vi "test2-ProcessSyncMessageInCSMLoop(SendAndReceive).vi"(8 "error in (no error)":errorcluster, 11 "TestCase in":refnum<class "testcase-CSMAddonLoopSupport.lvclass">) -> (0 "error out":errorcluster, 3 "TestCase out":refnum<class "testcase-CSMAddonLoopSupport.lvclass">)   [LabVIEW 2017, in "testcase-CSMAddonLoopSupport.lvclass"]
uses:
  testcase-CSMAddonLoopSupport.lvclass
  4585ddd5-ba69-4fd4-94fe-207595864cbd.vi
  a7620e19-6451-46a1-85ca-ade5edb58587.vi
  55fec5d7-cd22-46f7-b641-2c7c49619fc8.vi
  9cfd6824-310a-46c9-9b98-3854de5c7aa2.vi
  <vilib>/addons/_JKI Toolkits/VI Tester/TestCase.llb/TestCase.lvclass
  src/user.lib/_NEVSTOP/Communicable State Machine(CSM)/Communicable State Machine.lvlib
  C:/Program Files (x86)/National Instruments/LabVIEW 2017/vi.lib/addons/_JKI Toolkits/VI Tester/TestCase.llb/TestCase.lvclass
panel:
  out "LoopCount":i32
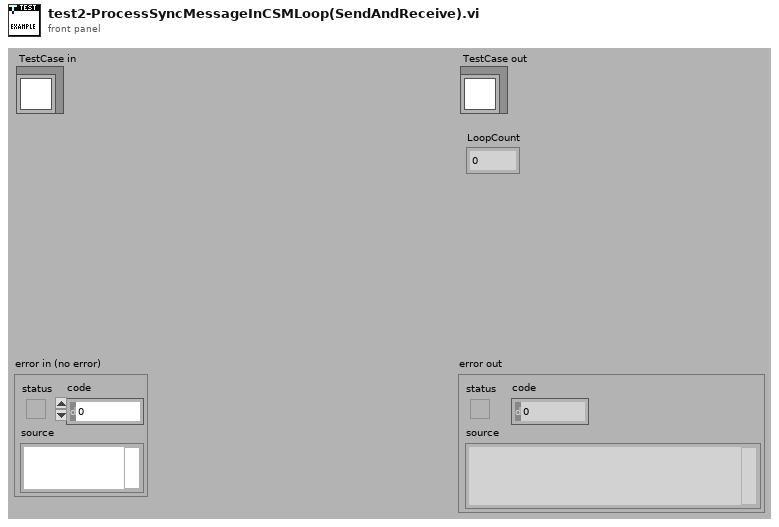
[diagram p1: front panel]
types:
  T1 = cluster{"Arguments":string, "Response":string, "error":errorcluster}
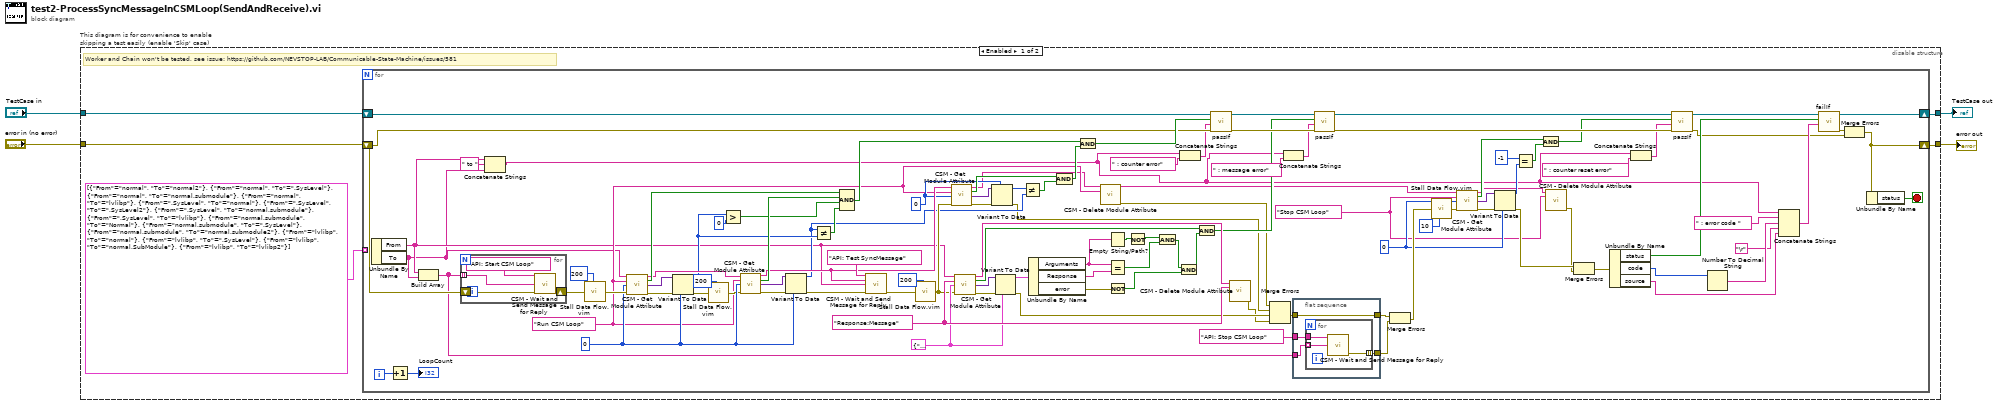
[diagram p0: block diagram]
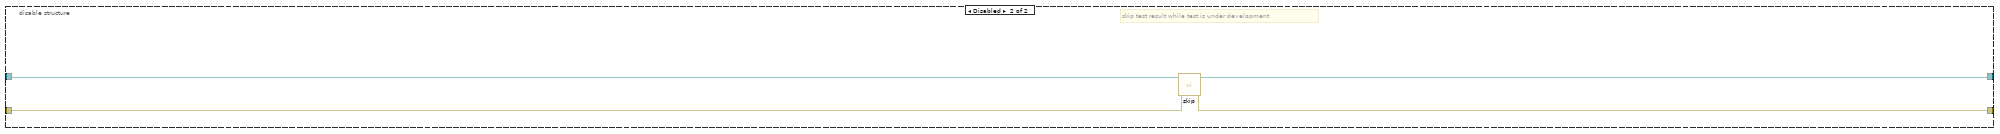
[diagram p2: hidden frame]
diagram:
  n1 = disable-structure "This diagram is for convenience to enable skipping a test easily (enable 'Skip' case)" shown="Enabled" {
    disable-tunnel: "TestCase in" -> [w9 w135]
    disable-tunnel: [w7 w133] -> w1
    disable-tunnel: [w6 w134] -> w3
    disable-tunnel: "error in (no error)" -> [w8 w132]
    frame Enabled {
      # "Worker and Chain won't be tested, see issue: https://github.com/NEVSTOP-LAB/Communicable-State-Machine/issues/581"
      n2 = for {
        tunnel: cluster{"From":string, "To":string}[] [{"From"="normal", "To"="normal2"}, {"From"="normal", "To"=".SysLevel"}, {"From"="normal", "To"="normal.submodule"}, {"From"="normal", "To"="lvlibp"}, {"From"=".SysLevel", "To"="normal"}, {"From"=".SysLevel", "To"=".SysLevel2"}, {"From"=".SysLevel", "To"="normal.submodule"}, {"From"=".SysLevel", "To"="lvlibp"}, {"From"="normal.submodule", "To"="Normal"}, {"From"="normal.submodule", "To"=".SysLevel"}, {"From"="normal.submodule", "To"="normal.submodule2"}, {"From"="lvlibp", "To"="normal"}, {"From"="lvlibp", "To"=".SysLevel"}, {"From"="lvlibp", "To"="normal.SubModule"}, {"From"="lvlibp", "To"="lvlibp2"}] -> [w30] mode=indexing
        shift-right: [w59] -> w7
        shift-left: w9 -> [w69]
        shift-right: [w11] -> w6
        shift-left: w8 -> [w60]
        i -> [w120]
        stop <- w63 stop-if-true
        w34 = "Stop CSM Loop" ("State")
        w47 = 0
        w72 = 0
        w87 = 0
        w38 = "Run CSM Loop" ("State")
        w98 = T1 {"Arguments"="", "Response"="", "error"={"status"=FALSE, "code"=0, "source"=""}}
        w99 = "Response:Message" ("State")
        n3 = Unbundle By Name(w30) -> ("From"=w28:string, "To"=w27:string)
        n4 = Increment(x=w120) -> (x+1=→"LoopCount":i32)
        n5 = Build Array(w28, w27) -> (w29:string[])
        n6 = for {
          shift-right: [w123] -> w118
          shift-left: w60 -> [w122]
          tunnel: w29 -> [w121] mode=indexing
          n7 = call "CSM - Wait and Send Message for Reply.vi"("State"="API: Start CSM Loop", "Target Module"=w121, "Error In (No Error)"=w122) -> ("error out"=w123:errorcluster)  [unwired: 9 in, 3 out]
        }
        n8 = Concatenate Strings(w28, " to " ("string"), w27) -> (w14:string)
        n9 = call "Stall Data Flow.vim"("value in"=w118, "milliseconds to wait"=u32 200) -> ("value out"=w95:errorcluster)  [unwired: 1 out]
        n10 = call "CSM - Get Module Attribute.vi"("CSM Name"=w27, "Attribute"=w38, "Default Value (Empty Variant)"=w87, "Error In"=w95) -> ("CSM Name (Dup)"=w89:string, "Found"=w94:bool, "Value"=w88:variant, "error out"=w92:errorcluster)  [unwired: 7 in, 1 out]
        n11 = Variant To Data(error in=w92, type=w87, Variant=w88) -> (data=w82:i32, error out=w81:errorcluster)
        n12 = call "Stall Data Flow.vim"("value in"=w81, "milliseconds to wait"=u32 200) -> ("value out"=w80:errorcluster)  [unwired: 1 out]
        n13 = Greater?(x=w82, y=0) -> (0:w85:bool)
        n14 = call "CSM - Get Module Attribute.vi"("CSM Name"=w89, "Attribute"=w38, "Default Value (Empty Variant)"=w87, "Error In"=w80) -> ("CSM Name (Dup)"=w77:string, "Found"=w93:bool, "Value"=w84:variant, "error out"=w91:errorcluster)  [unwired: 7 in, 1 out]
        n15 = Variant To Data(error in=w91, type=w87, Variant=w84) -> (data=w70:i32, error out=w90:errorcluster)
        n16 = Not Equal?(x=w70, y=w82) -> (x != y?=w83:bool)
        n17 = Compound Arithmetic op=AND(w94, w93, w85, w83) -> (w68:bool)
        n18 = call "CSM - Wait and Send Message for Reply.vi"("State"="API: Test SyncMessage", "Arguments (\"\")"=w77, "Target Module"=w28, "Error In (No Error)"=w90) -> ("error out"=w114:errorcluster)  [unwired: 8 in, 3 out]
        n19 = call "Stall Data Flow.vim"("value in"=w114, "milliseconds to wait"=u32 200) -> ("value out"=w78:errorcluster)  [unwired: 1 out]
        n20 = call "CSM - Get Module Attribute.vi"("CSM Name"=w77, "Attribute"=w38, "Default Value (Empty Variant)"=w72, "Error In"=w78) -> ("CSM Name (Dup)"=w37:string, "Found"=w74:bool, "Value"=w73:variant, "error out"=w75:errorcluster)  [unwired: 7 in, 1 out]
        n21 = call "CSM - Get Module Attribute.vi"("CSM Name"=w28, "Attribute"=w99, "Default Value (Empty Variant)"=w98, "Error In"=w78) -> ("CSM Name (Dup)"=w107:string, "Found"=w109:bool, "Value"=w112:variant, "error out"=w113:errorcluster)  [unwired: 7 in, 1 out]
        n22 = Variant To Data(error in=w75, type=w72, Variant=w73) -> (data=w71:i32, error out=w36:errorcluster)
        n23 = Variant To Data(error in=w113, type=w98, Variant=w112) -> (data=w111:T1, error out=w97:errorcluster)
        n24 = Not Equal?(x=w71, y=w70) -> (x != y?=w76:bool)
        n25 = Unbundle By Name(w111) -> ("Arguments"=w102:string, "Response"=w101:string, "error"=w100:errorcluster)
        n26 = Compound Arithmetic op=AND(w74, w76) -> (w67:bool)
        n27 = And(x=w68, y=w67) -> (x .and. y?=w66:bool)
        n28 = call "CSM - Delete Module Attribute.vi"("CSM Name"=w37, "Attribute"=w38) -> ("CSM Name (Dup)"=w33:string, "error out"=w35:errorcluster)  [unwired: 10 in, 2 out]
        n29 = Empty String/Path?(string/path=w102) -> (empty?=w106:bool)
        n30 = Equal?(x=w102, y=w101) -> (x = y?=w104:bool)
        n31 = Not(x=w100) -> (.not. x?=w110:bool)
        n32 = Not(x=w106) -> (.not. x?=w105:bool)
        n33 = And(x=w105, y=w104) -> (x .and. y?=w103:bool)
        n34 = And(x=w103, y=w110) -> (x .and. y?=w108:bool)
        n35 = Concatenate Strings(w14, " : counter error" ("format string")) -> (w24:string)
        n36 = And(x=w109, y=w108) -> (x .and. y?=w62:bool)
        n37 = call-dynamic "passIf.vi"("error in (no error)"=w60, "message (\"\")"=w24, "pass"=w66, "TestCase in"=w69) -> ("error out"=w64:errorcluster, "TestCase out"=w65:refnum<class "testcase-CSMAddonLoopSupport.lvclass">)  [unwired: 6 in]
        n38 = call "CSM - Delete Module Attribute.vi"("CSM Name"=w107, "Attribute"=w99) -> ("error out"=w96:errorcluster)  [unwired: 10 in, 3 out]
        n39 = Merge Errors(w35, w36, w97, w96) -> (w39:errorcluster)
        n40 = Concatenate Strings(w14, " : message error" ("format string")) -> (w22:string)
        n41 = flat-sequence {
          tunnel: "API: Stop CSM Loop" ("State") -> [w128]
          tunnel: [w127] -> w54
          tunnel: [w126] -> w40
          tunnel: w39 -> [w126]
          tunnel: w29 -> [w125]
          frame #0 {
            n42 = for {
              tunnel: w128 -> [w131]
              tunnel: [w130] -> w127 mode=indexing
              tunnel: w125 -> [w129] mode=indexing
              n43 = call "CSM - Wait and Send Message for Reply.vi"("State"=w131, "Target Module"=w129) -> ("error out"=w130:errorcluster)  [unwired: 10 in, 3 out]
            }
          }
        }
        n44 = call-dynamic "passIf.vi"("error in (no error)"=w64, "message (\"\")"=w22, "pass"=w62, "TestCase in"=w65) -> ("error out"=w55:errorcluster, "TestCase out"=w57:refnum<class "testcase-CSMAddonLoopSupport.lvclass">)  [unwired: 6 in]
        n45 = Merge Errors(w40, w54) -> (w52:errorcluster)
        n46 = call "Stall Data Flow.vim"("value in"=w52, "milliseconds to wait"=u32 10) -> ("value out"=w51:errorcluster)  [unwired: 1 out]
        n47 = call "CSM - Get Module Attribute.vi"("CSM Name"=w33, "Attribute"=w34, "Default Value (Empty Variant)"=w47, "Error In"=w51) -> ("CSM Name (Dup)"=w32:string, "Found"=w50:bool, "Value"=w48:variant, "error out"=w49:errorcluster)  [unwired: 7 in, 1 out]
        n48 = Variant To Data(error in=w49, type=w47, Variant=w48) -> (data=w46:i32, error out=w42:errorcluster)
        n49 = Equal?(x=-1, y=w46) -> (x = y?=w43:bool)
        n50 = And(x=w50, y=w43) -> (x .and. y?=w44:bool)
        n51 = call "CSM - Delete Module Attribute.vi"("CSM Name"=w32, "Attribute"=w34) -> ("error out"=w41:errorcluster)  [unwired: 10 in, 3 out]
        n52 = Merge Errors(w42, w41) -> (w31:errorcluster)
        n53 = Unbundle By Name(w31) -> ("status"=w19:bool, "code"=w13:i32, "source"=w12:string)
        n54 = Concatenate Strings(w14, " : counter reset error" ("format string")) -> (w20:string)
        n55 = call-dynamic "passIf.vi"("error in (no error)"=w55, "message (\"\")"=w20, "pass"=w44, "TestCase in"=w57) -> ("error out"=w10:errorcluster, "TestCase out"=w56:refnum<class "testcase-CSMAddonLoopSupport.lvclass">)  [unwired: 6 in]
        n56 = Number To Decimal String(number=w13) -> (decimal integer string=w17:string)  [unwired: 1 in]
        n57 = Concatenate Strings(w14, " : error code " ("format string"), w17, "\r", w12) -> (w15:string)
        n58 = call-dynamic "failIf.vi"("message (\"\")"=w15, "fail"=w19, "TestCase in"=w56) -> ("error out"=w58:errorcluster, "TestCase out"=w59:refnum<class "testcase-CSMAddonLoopSupport.lvclass">)  [unwired: 7 in]
        n59 = Merge Errors(w58, w10) -> (w11:errorcluster)
        n60 = Unbundle By Name(w11) -> ("status"=w63:bool)
      }
    }
    frame Disabled {
      # "skip test result while test is under development"
      n61 = call <vilib>:"skip.vi"("error in (no error)"=w132, "TestCase in"=w135) -> ("error out"=w134:errorcluster, "TestCase out"=w133:refnum<class "testcase-CSMAddonLoopSupport.lvclass">)  [unwired: 8 in]
    }
  }
  "error out" <- w3
  "TestCase out" <- w1
